vi "Margins.vi"(8 "error in (no error)":errorcluster, 10 "Page setup IN":T1={"Page Size"=1, "Orientation"=enum."Portrait", "Custom Layout"={"Width"=0.0, "Height"=0.0}, "Margins"={"Left"=25.0, "Right"=25.0, "Top"=25.0, "Bottom"=25.0}} {"Page Size" items=["Custom", "LETTER", "NOTE", "LEGAL", "TABLOID", "EXECUTIVE", "POSTCARD", "A0", "A1", "A2", "A3", "A4", "A5", "A6", "A7", "A8", "A9", "A10", "B0", "B1", "B2", "B3", "B4", "B5", "B6", "B7", "B8", "B9", "B10", "ARCH_E", "ARCH_D", "ARCH_C", "ARCH_B", "ARCH_A", "FLSA", "FLSE", "HALFLETTER", "_11X17", "ID_1", "ID_2", "ID_3", "LEDGER", "CROWN_QUARTO", "LARGE_CROWN_QUARTO", "DEMY_QUARTO", "ROYAL_QUARTO", "CROWN_OCTAVO", "LARGE_CROWN_OCTAVO", "DEMY_OCTAVO", "ROYAL_OCTAVO", "SMALL_PAPERBACK", "PENGUIN_SMALL_PAPERBACK", "PENGUIN_LARGE_PAPERBACK"]}, 11 "Unit (default = mm)":T6=enum."mm") -> (0 "error out":errorcluster, 2 "Page setup OUT":T1={"Page Size"=1, "Orientation"=enum."Portrait", "Custom Layout"={"Width"=0.0, "Height"=0.0}, "Margins"={"Left"=25.0, "Right"=25.0, "Top"=25.0, "Bottom"=25.0}} {"Page Size" items=["Custom", "LETTER", "NOTE", "LEGAL", "TABLOID", "EXECUTIVE", "POSTCARD", "A0", "A1", "A2", "A3", "A4", "A5", "A6", "A7", "A8", "A9", "A10", "B0", "B1", "B2", "B3", "B4", "B5", "B6", "B7", "B8", "B9", "B10", "ARCH_E", "ARCH_D", "ARCH_C", "ARCH_B", "ARCH_A", "FLSA", "FLSE", "HALFLETTER", "_11X17", "ID_1", "ID_2", "ID_3", "LEDGER", "CROWN_QUARTO", "LARGE_CROWN_QUARTO", "DEMY_QUARTO", "ROYAL_QUARTO", "CROWN_OCTAVO", "LARGE_CROWN_OCTAVO", "DEMY_OCTAVO", "ROYAL_OCTAVO", "SMALL_PAPERBACK", "PENGUIN_SMALL_PAPERBACK", "PENGUIN_LARGE_PAPERBACK"]}, 3 "Rectangle":refnum<k24>)   [LabVIEW 2012]
doc: "Version 1.0\nDeveloped by Jean-Marc Simard\nCopyright © 2010, Exaprom Inc.\nAll rights reserved.\nLicense: BSD\n\nWith iTextSharp 4.1.6 (http://itextsharp.sourceforge.net)\nunder Mozilla Public License Version 1.1\n(http://www.mozilla.org/MPL/MPL-1.1.html)"
uses:
  Controls/Page setup.ctl
  Controls/Page size.ctl
  Controls/Page Orientation.ctl
  Controls/Page Layout Custom.ctl
  Controls/Page margins.ctl
  Controls/Unit.ctl
  C:/Users/MaxCorp/Documents/TopPerm - Base/DLL/itextsharp.dll
  DLL/itextsharp.dll
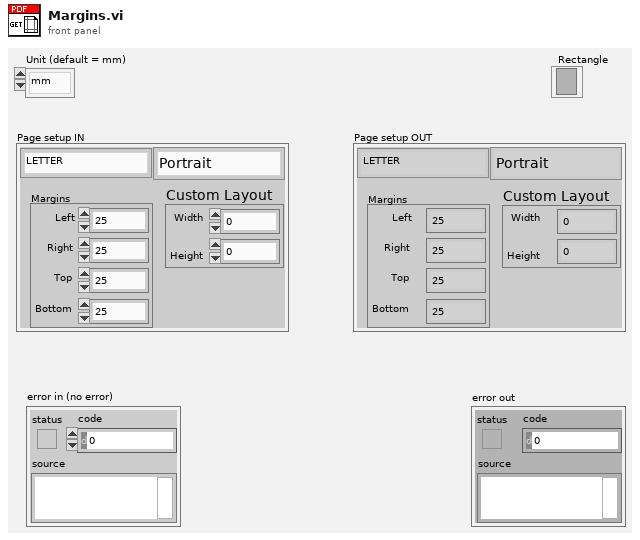
[diagram p1: front panel]
types:
  T1 = typedef "Page setup.ctl" = cluster{"Page Size":T2, "Orientation":T3, "Custom Layout":T4, "Margins":T5}
  T2 = typedef "Page size.ctl" = i32
  T3 = typedef "Page Orientation.ctl" = enum16{"Portrait", "Landscape"}
  T4 = typedef "Page Layout Custom.ctl" = cluster{"Width":sgl, "Height":sgl}
  T5 = typedef "Page margins.ctl" = cluster{"Left":sgl, "Right":sgl, "Top":sgl, "Bottom":sgl}
  T6 = typedef "Unit.ctl" = enum16{"inch", "mm"}
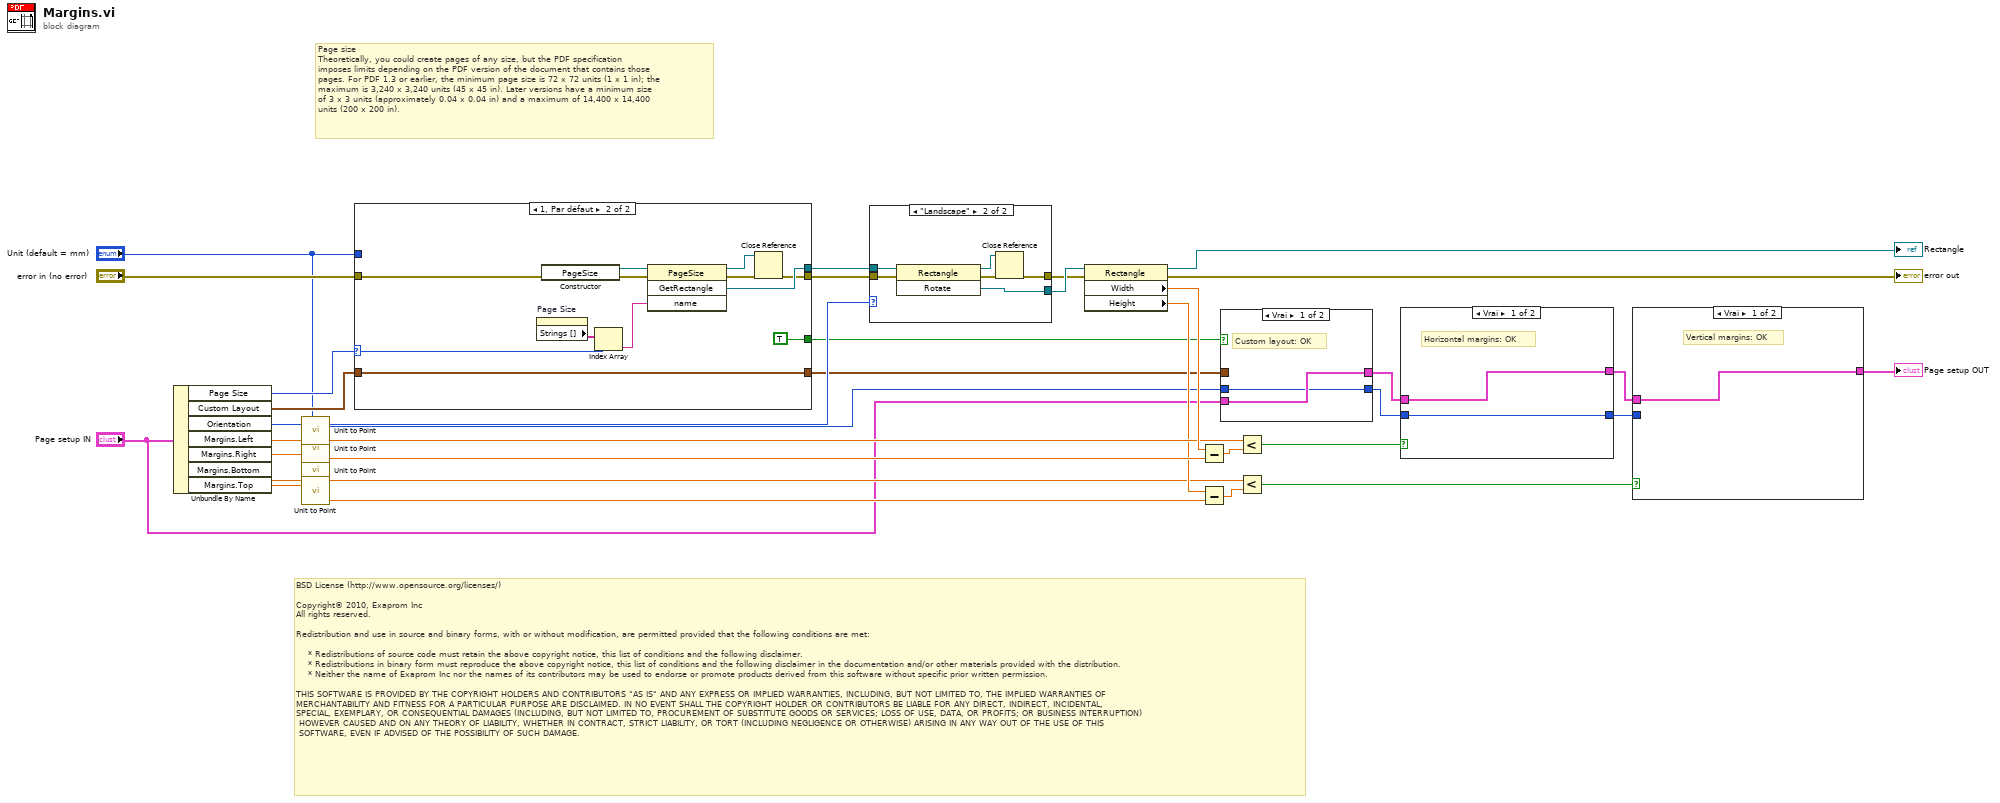
[diagram p0: block diagram]
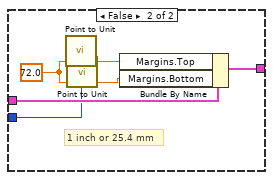
[diagram p2: hidden frame]
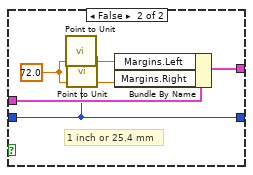
[diagram p3: hidden frame]
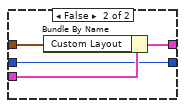
[diagram p4: hidden frame]
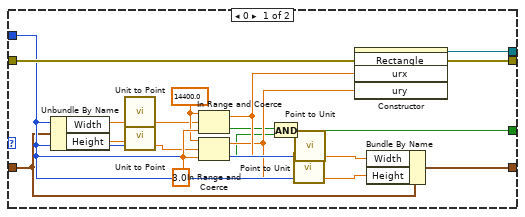
[diagram p6: hidden frame]
diagram:
  # "BSD License (http://www.opensource.org/licenses/)\n\nCopyright© 2010, Exaprom Inc\nAll rights reserved.\n\nRedistribution and use in source and binary forms, with or without modification, are permitted provided that the following conditions are met:\n\n    * Redistributions of source code must retain the above copyright notice, this list of conditions and the following disclaimer.\n    * Redistributions in binary form must reproduce the above copyright notice, this list of conditions and the following disclaimer in the documentation and/or other materials provided with the distribution.\n    * Neither the name of Exaprom Inc nor the names of its contributors may be used to endorse or promote products derived from this software without specific prior written permission.\n\nTHIS SOFTWARE IS PROVIDED BY THE COPYRIGHT HOLDERS AND CONTRIBUTORS \"AS IS\" AND ANY EXPRESS OR IMPLIED WARRANTIES, INCLUDING, BUT NOT LIMITED TO, THE IMPLIED WARRANTIES OF \nMERCHANTABILITY AND FITNESS FOR A PARTICULAR PURPOSE ARE DISCLAIMED. IN NO EVENT SHALL THE COPYRIGHT HOLDER OR CONTRIBUTORS BE LIABLE FOR ANY DIRECT, INDIRECT, INCIDENTAL,\nSPECIAL, EXEMPLARY, OR CONSEQUENTIAL DAMAGES (INCLUDING, BUT NOT LIMITED TO, PROCUREMENT OF SUBSTITUTE GOODS OR SERVICES; LOSS OF USE, DATA, OR PROFITS; OR BUSINESS INTERRUPTION)\n HOWEVER CAUSED AND ON ANY THEORY OF LIABILITY, WHETHER IN CONTRACT, STRICT LIABILITY, OR TORT (INCLUDING NEGLIGENCE OR OTHERWISE) ARISING IN ANY WAY OUT OF THE USE OF THIS\n SOFTWARE, EVEN IF ADVISED OF THE POSSIBILITY OF SUCH DAMAGE."
  # "Page size\nTheoretically, you could create pages of any size, but the PDF specification\nimposes limits depending on the PDF version of the document that contains those\npages. For PDF 1.3 or earlier, the minimum page size is 72 x 72 units (1 x 1 in); the\nmaximum is 3,240 x 3,240 units (45 x 45 in). Later versions have a minimum size\nof 3 x 3 units (approximately 0.04 x 0.04 in) and a maximum of 14,400 x 14,400\nunits (200 x 200 in)."
  n1 = Unbundle By Name("Page setup IN") -> ("Page Size"=w33:T2, "Custom Layout"=w32:T4, "Orientation"=w26:T3, "Margins.Left"=w30:sgl, "Margins.Right"=w29:sgl, "Margins.Bottom"=w28:sgl, "Margins.Top"=w27:sgl)
  n2 = call "Unit to Point.vi"("X unit"=w30, "Unit (default = mm)"="Unit (default = mm)") -> ("X point"=w19:sgl)  [unwired: 7 out]
  n3 = call "Unit to Point.vi"("X unit"=w29, "Unit (default = mm)"="Unit (default = mm)") -> ("X point"=w20:sgl)  [unwired: 7 out]
  n4 = call "Unit to Point.vi"("X unit"=w28, "Unit (default = mm)"="Unit (default = mm)") -> ("X point"=w16:sgl)  [unwired: 7 out]
  n5 = call "Unit to Point.vi"("X unit"=w27, "Unit (default = mm)"="Unit (default = mm)") -> ("X point"=w15:sgl)  [unwired: 7 out]
  n6 = case shown="1, Par défaut" w33 {
    selector: w33 -> [_ w61]
    tunnel: [w52 w56] -> w31
    tunnel: [w51 w64] -> w1
    tunnel: w32 -> [w37 w54]
    tunnel: "error in (no error)" -> [w50 w55]
    tunnel: "Unit (default = mm)" -> [w43 _]
    tunnel: [w38 w54] -> w13
    tunnel: [w34 TRUE] -> w12
    frame 0 {
      w48 = sgl 14400.0
      w49 = sgl 3.0
      n7 = Unbundle By Name(w37) -> ("Width"=w47:sgl, "Height"=w46:sgl)
      n8 = call "Unit to Point.vi"("X unit"=w47, "Unit (default = mm)"=w43) -> ("X point"=w44:sgl)  [unwired: 7 out]
      n9 = call "Unit to Point.vi"("X unit"=w46, "Unit (default = mm)"=w43) -> ("X point"=w45:sgl)  [unwired: 7 out]
      n10 = In Range and Coerce(upper limit=w48, x=w44, lower limit=w49) -> (coerced(x)=w42:sgl, In Range?=w36:bool)
      n11 = In Range and Coerce(upper limit=w48, x=w45, lower limit=w49) -> (coerced(x)=w41:sgl, In Range?=w35:bool)
      n12 = And(x=w36, y=w35) -> (x .and. y?=w34:bool)
      n13 = call "Point to Unit.vi"("X point"=w41, "Unit (default = mm)"=w43) -> ("X unit"=w39:sgl)  [unwired: 7 out]
      n14 = call "Point to Unit.vi"("X point"=w42, "Unit (default = mm)"=w43) -> ("X unit"=w40:sgl)  [unwired: 7 out]
      n15 = constructor class="Rectangle"(error in=w50, "urx"=w42, "ury"=w41) -> (reference out=w51:refnum<k24>, error out=w52:errorcluster)  [unwired: 2 in, 3 out]
      n16 = Bundle By Name(cluster=w37, "Width"=w40, "Height"=w39) -> (w38:T4)
    }
    frame 1, Default {
      n17 = property on="Page Size" class="MDér (strict)"() -> ("Strings []"=w62:string[])  [unwired: 2 in, 2 out]
      n18 = constructor class="PageSize"(error in=w55) -> (reference out=w60:refnum<k24>, error out=w59:errorcluster)  [unwired: 2 in, 1 out]
      n19 = Index Array(array=w62, index=w61) -> (element=w63:string)
      n20 = invoke class="PageSize" method="GetRectangle"(reference=w60, error in=w59, "name"=w63) -> (reference out=w57:refnum<k24>, error out=w58:errorcluster, "GetRectangle"=w64:refnum<k24>)  [unwired: 1 in, 1 out]
      n21 = Close Reference(reference=w57, error in (no error)=w58) -> (error out=w56:errorcluster)
    }
  }
  n22 = case shown="\"Landscape\"" w26 {
    tunnel: [w65 w67] -> w22
    tunnel: [w66 w72] -> w25
    tunnel: w1 -> [w66 w71]
    tunnel: w31 -> [w65 w70]
    frame "Portrait", Default {
    }
    frame "Landscape" {
      n23 = invoke class="Rectangle" method="Rotate"(reference=w71, error in=w70) -> (reference out=w68:refnum<k24>, error out=w69:errorcluster, "Rotate"=w72:refnum<k24>)  [unwired: 1 in]
      n24 = Close Reference(reference=w68, error in (no error)=w69) -> (error out=w67:errorcluster)
    }
  }
  n25 = property class="Rectangle"(reference=w25, error in=w22) -> (reference out=→"Rectangle":refnum<k24>, error out=→"error out":errorcluster, "Width"=w21:sgl, "Height"=w17:sgl)
  n26 = Subtract(x=w21, y=w20) -> (x-y=w18:sgl)
  n27 = Subtract(x=w17, y=w15) -> (x-y=w14:sgl)
  n28 = case shown="Vrai" w12 {
    tunnel: [w74 w78] -> w8
    tunnel: w13 -> [_ w77]
    tunnel: "Unit (default = mm)" -> [w73 w75]
    tunnel: "Page setup IN" -> [w74 w76]
    tunnel: [w73 w75] -> w7
    frame True {
      # "Custom layout: OK"
    }
    frame False {
      n29 = Bundle By Name(cluster=w76, "Custom Layout"=w77) -> (w78:T1)
    }
  }
  n30 = Less?(x=w19, y=w18) -> (x < y?=w9:bool)
  n31 = Less?(x=w16, y=w14) -> (x < y?=w3:bool)
  n32 = case shown="Vrai" w9 {
    tunnel: [w80 w83] -> w5
    tunnel: w8 -> [w80 w82]
    tunnel: w7 -> [w79 w81]
    tunnel: [w79 w81] -> w6
    frame True {
      # "Horizontal margins: OK"
    }
    frame False {
      w86 = sgl 72.0 ("X point")
      # "1 inch or 25.4 mm"
      n33 = call "Point to Unit.vi"("X point"=w86, "Unit (default = mm)"=w81) -> ("X unit"=w84:sgl)  [unwired: 7 out]
      n34 = call "Point to Unit.vi"("X point"=w86, "Unit (default = mm)"=w81) -> ("X unit"=w85:sgl)  [unwired: 7 out]
      n35 = Bundle By Name(cluster=w82, "Margins.Left"=w84, "Margins.Right"=w85) -> (w83:T1)
    }
  }
  n36 = case shown="Vrai" w3 {
    tunnel: [w87 w90] -> w4
    tunnel: w5 -> [w87 w89]
    tunnel: w6 -> [_ w88]
    frame True {
      # "Vertical margins: OK"
    }
    frame False {
      w93 = sgl 72.0 ("X point")
      # "1 inch or 25.4 mm"
      n37 = call "Point to Unit.vi"("X point"=w93, "Unit (default = mm)"=w88) -> ("X unit"=w91:sgl)  [unwired: 7 out]
      n38 = call "Point to Unit.vi"("X point"=w93, "Unit (default = mm)"=w88) -> ("X unit"=w92:sgl)  [unwired: 7 out]
      n39 = Bundle By Name(cluster=w89, "Margins.Top"=w91, "Margins.Bottom"=w92) -> (w90:T1)
    }
  }
  "Page setup OUT" <- w4
